vi "Send Error Warning.vi"(4 "Message Body":string="The is a possible problem.", 5 "Contact":T1, 6 "Message Subject":string="Check the Laser!", 7 "Action on Error":T2(ring), 8 "error in":errorcluster, 9 "Email Password":string="apatite2Z", 10 "Email Username":string="raymond.apatite@gmail.com", 11 "SMTP Server":string="smtp.gmail.com") -> (0 "error out":errorcluster)   [LabVIEW 2013]
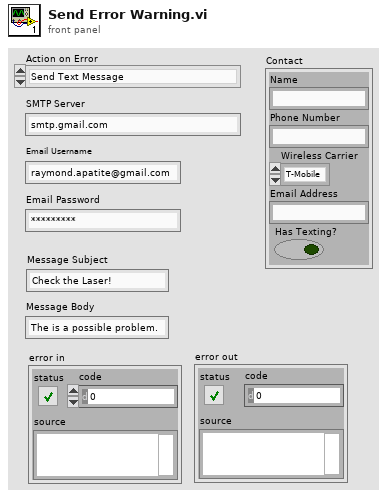
[diagram p1: front panel]
types:
  T1 = cluster{"Name":string, "Phone Number":string, "Wireless Carrier":enum16{"T-Mobile", "AT&T", "Verizon", "Sprint"}, "Email Address":string, "Has Texting?":bool}
  T2 = enum16{"Send Text Message", "Send Email", "Send Text Message & Email"}
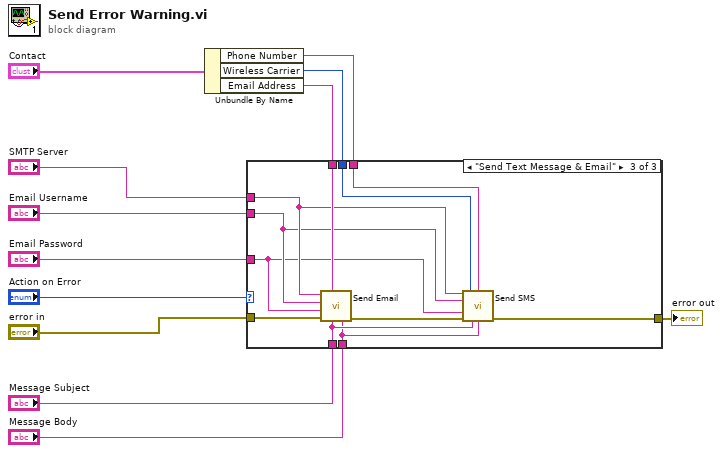
[diagram p0: block diagram]
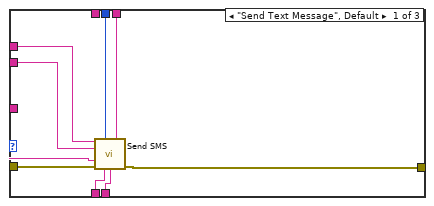
[diagram p2: hidden frame]
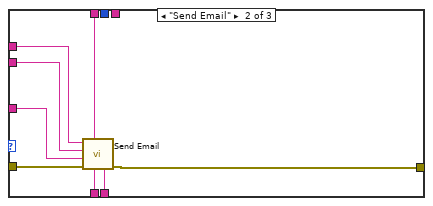
[diagram p3: hidden frame]
diagram:
  n1 = Unbundle By Name("Contact") -> ("Phone Number"=w12:string, "Wireless Carrier"=w11:enum16{"T-Mobile", "AT&T", "Verizon", "Sprint"}, "Email Address"=w10:string)
  n2 = case shown="\"Send Text Message & Email\"" "Action on Error" {
    tunnel: "error in" -> [w16 w29 w40]
    tunnel: [w13 w23 w30] -> w1
    tunnel: "Message Subject" -> [w15 w28 w32]
    tunnel: "Message Body" -> [w14 w27 w31]
    tunnel: "SMTP Server" -> [w19 w26 w36]
    tunnel: "Email Username" -> [w18 w25 w35]
    tunnel: "Email Password" -> [w17 w24 w34]
    tunnel: w10 -> [_ w22 w39]
    tunnel: w11 -> [w20 _ w37]
    tunnel: w12 -> [w21 _ w38]
    frame "Send Text Message", Default {
      n3 = call "Send SMS.vi"("SMTP Server"=w19, "Carrier"=w20, "Phone Number"=w21, "Email Username"=w18, "Email Password"=w17, "error in (no error)"=w16, "Subject"=w15, "Body"=w14) -> ("error out"=w13:errorcluster)  [unwired: 7 in]
    }
    frame "Send Email" {
      n4 = call "Send Email.vi"("Body"=w27, "Subject"=w28, "Email Address"=w22, "error in (no error)"=w29, "Email Password"=w24, "Email Username"=w25, "SMTP Server"=w26) -> ("error out"=w23:errorcluster)  [unwired: 4 in]
    }
    frame "Send Text Message & Email" {
      n5 = call "Send Email.vi"("Body"=w31, "Subject"=w32, "Email Address"=w39, "error in (no error)"=w40, "Email Password"=w34, "Email Username"=w35, "SMTP Server"=w36) -> ("error out"=w33:errorcluster)  [unwired: 4 in]
      n6 = call "Send SMS.vi"("SMTP Server"=w36, "Carrier"=w37, "Phone Number"=w38, "Email Username"=w35, "Email Password"=w34, "error in (no error)"=w33, "Subject"=w32, "Body"=w31) -> ("error out"=w30:errorcluster)  [unwired: 7 in]
    }
  }
  "error out" <- w1
